vi "MatchFormatString.vi"(10 "Input String":string, 11 "Format String":string) -> (2 "Match Found?":bool, 3 "Tag Map":map{string, string}(c390))   [LabVIEW 2019, in "LabErrorUX.lvclass"]
uses:
  LabErrorUX.lvclass
  <vilib>/regexp/Match Regular Expression.xnode
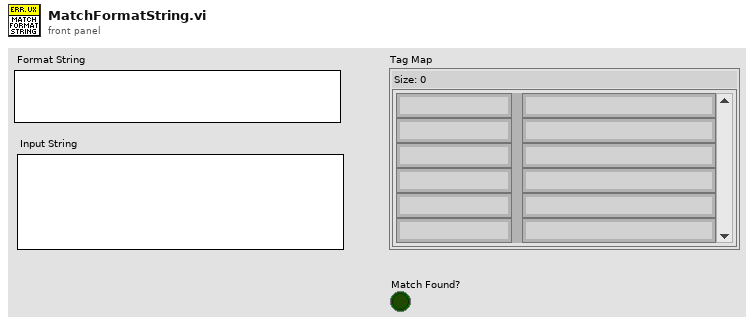
[diagram p1: front panel]
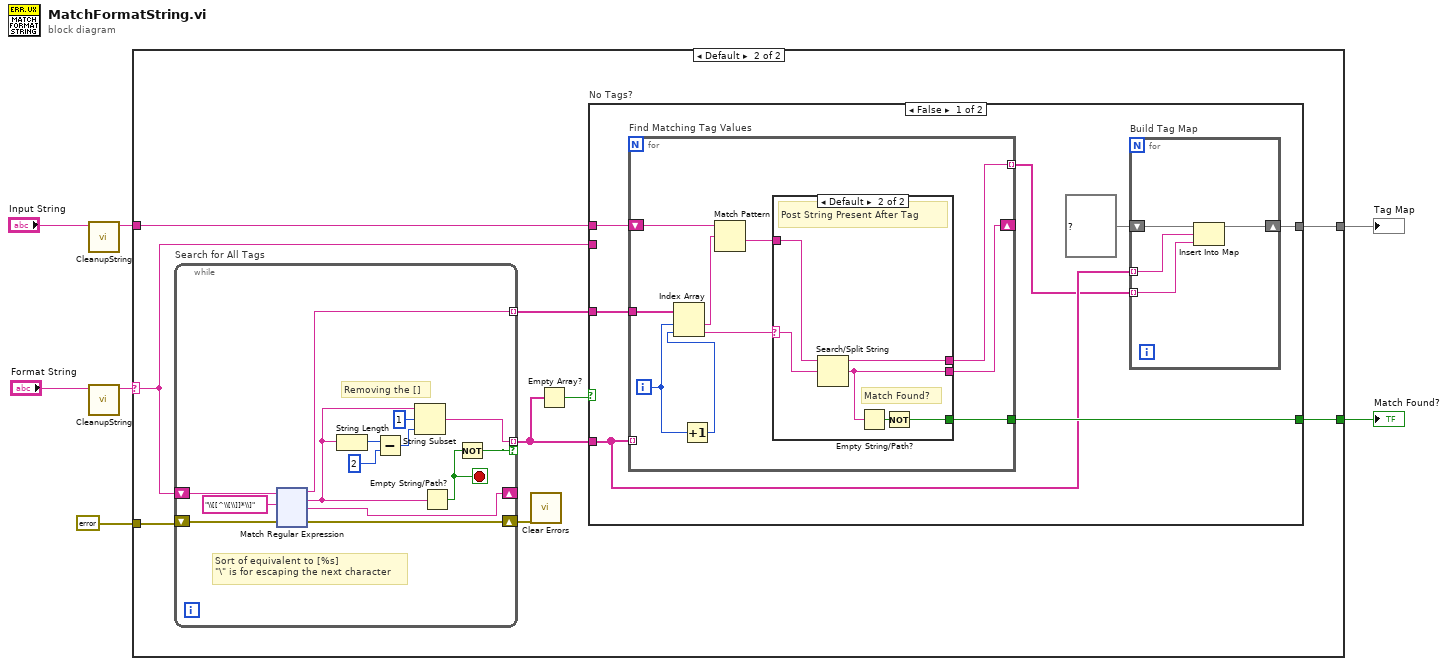
[diagram p0: block diagram]
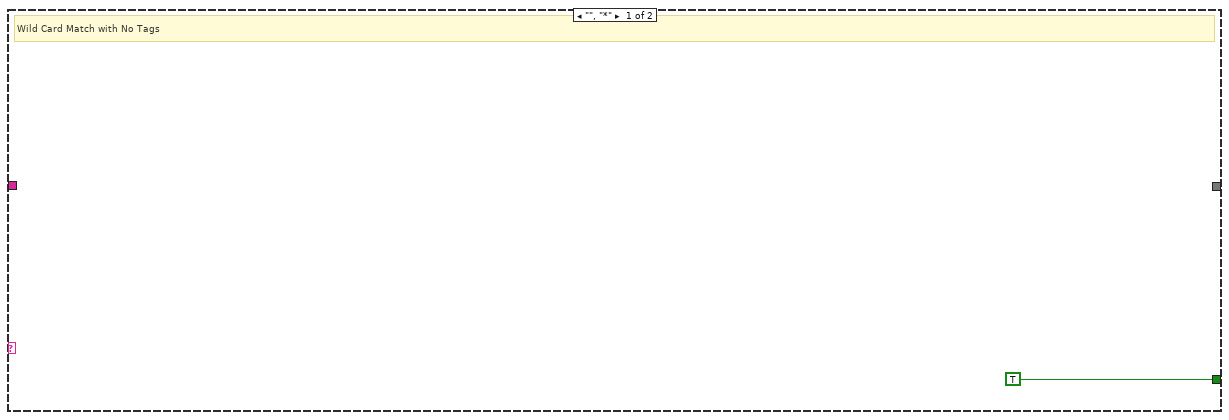
[diagram p2: hidden frame]
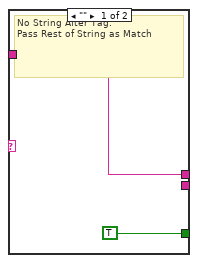
[diagram p3: hidden frame]
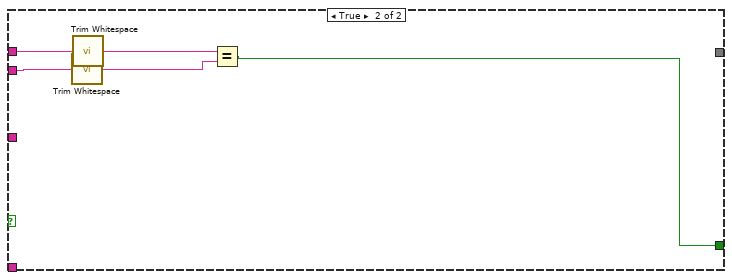
[diagram p4: hidden frame]
diagram:
  n1 = call "CleanupString.vi"("Input String"="Input String") -> ("Output String"=w4:string)  [unwired: 10 in]
  n2 = call "CleanupString.vi"("Input String"="Format String") -> ("Output String"=w1:string)  [unwired: 10 in]
  n3 = case shown="Default" w1 {
    selector: w1 -> [_ w9]
    tunnel: w4 -> [_ w17]
    tunnel: [TRUE w15] -> w7
    tunnel: [_ w14] -> w6
    tunnel: errorcluster {"status"=FALSE, "code"=0, "source"=""} ("error in") -> [_ w13]
    frame "", "*" {
      # "Wild Card Match with No Tags"
    }
    frame Default {
      n4 = while "Search for All Tags" {
        shift-right: [w63] -> w12
        shift-left: w13 -> [w64]
        tunnel: [w59] -> w11 mode=indexing if=w60
        tunnel: [w53] -> w16 mode=indexing
        shift-right: [w52] -> _
        shift-left: w9 -> [w65]
        stop <- w61 stop-if-true
        # "Removing the []"
        # "Sort of equivalent to [%s]\n\"\\\" is for escaping the next character"
        n5 = xnode "Match Regular Expression"("input string"=w65, "regular expression"="\\[[^\\[\\]]*\\]", "error in"=w64) -> ("before match"=w53:string, "whole match"=w57:string, "after match"=w52:string, "error out"=w63:errorcluster)  [unwired: 3 in, 1 out]
        n6 = String Length(string=w57) -> (length=w56:i32)
        n7 = Subtract(x=w56, y=2) -> (x-y=w54:i32)
        n8 = String Subset(string=w57, offset (0)=1, length (rest)=w54) -> (substring=w59:string)
        n9 = Empty String/Path?(string/path=w57) -> (empty?=w61:bool)
        n10 = Not(x=w61) -> (.not. x?=w60:bool)
      }
      n11 = call <vilib>:"Clear Errors.vi"("error in (no error)"=w12) -> ()  [unwired: 5 in, 2 out]
      n12 = Empty Array?(array=w11) -> (empty?=w10:bool)
      n13 = case "No Tags?" shown="False" w10 {
        tunnel: w17 -> [w24 w51]
        tunnel: w16 -> [w23 _]
        tunnel: [w22 w47] -> w15
        tunnel: w11 -> [w21 _]
        tunnel: [w18 _] -> w14
        tunnel: w9 -> [_ w50]
        frame False {
          n14 = for "Find Matching Tag Values" {
            tunnel: w23 -> [w37]
            shift-right: [w32] -> _
            shift-left: w24 -> [w38]
            tunnel: [w33] -> w20 mode=indexing
            tunnel: w21 -> [_] mode=indexing
            tunnel: [w29] -> w22
            i -> [w36]
            n15 = Increment(x=w36) -> (x+1=w31:i32)
            n16 = Index Array(array=w37, index #1=w36, index #2=w31) -> (element #1=w35:string, element #2=w30:string)
            n17 = Match Pattern(string=w38, regular expression=w35) -> (after substring=w34:string)  [unwired: 1 in, 3 out]
            n18 = case shown="Default" w30 {
              selector: w30 -> [_ w45]
              tunnel: w34 -> [w40 w46]
              tunnel: [_ w42] -> w32
              tunnel: [w40 w44] -> w33
              tunnel: [TRUE w41] -> w29
              frame "" {
                # "No String After Tag.\nPass Rest of String as Match"
              }
              frame Default {
                # "Match Found?"
                # "Post String Present After Tag"
                n19 = Search/Split String(string=w46, search string/char (-)=w45) -> (substring before match=w44:string, match + rest of string=w42:string)  [unwired: 1 in, 1 out]
                n20 = Empty String/Path?(string/path=w42) -> (empty?=w43:bool)
                n21 = Not(x=w43) -> (.not. x?=w41:bool)
              }
            }
          }
          n22 = for "Build Tag Map" {
            tunnel: w21 -> [w26] mode=indexing
            tunnel: w20 -> [w25] mode=indexing
            shift-right: [w27] -> w18
            shift-left: map{string, string} {} ("map") -> [w28]
            n23 = Insert Into Map(map in=w28, key=w26, value=w25) -> (map out=w27:map{string, string})  [unwired: 2 out]
          }
        }
        frame True {
          n24 = call <vilib>:"Trim Whitespace.vi"("string"=w50) -> ("trimmed string"=w48:string)  [unwired: 1 in]
          n25 = call <vilib>:"Trim Whitespace.vi"("string"=w51) -> ("trimmed string"=w49:string)  [unwired: 1 in]
          n26 = Equal?(x=w49, y=w48) -> (x = y?=w47:bool)
        }
      }
    }
  }
  "Match Found?" <- w7
  "Tag Map" <- w6
